vi "Motor Waveforms.vi"(10 "Log Data in":cluster{refnum<class "RDS State.lvclass">[]}[](array[cluster]), 11 "Log Header In":T1) -> (2 "Log Data out":cluster{refnum<class "RDS State.lvclass">[]}[](array[cluster]), 3 "Log Header Out":T1, 5 "STBD Motor WFs":waveform(dbl)[](array[waveform]), 7 "Port Motor WFs":waveform(dbl)[](array[waveform]))   [LabVIEW 2015, in "Log Waveform Processors.lvlib"]
uses:
  Log Waveform Processors.lvlib
  RDS State Tracker/RDS State/RDS State.lvclass
  Actors/RDS Logger Actor/RDS Logger Actor/RDS Logger Actor/Logger Header.ctl
  RDS State Tracker/RDS State/RDS State.lvclass/RDS State.ctl
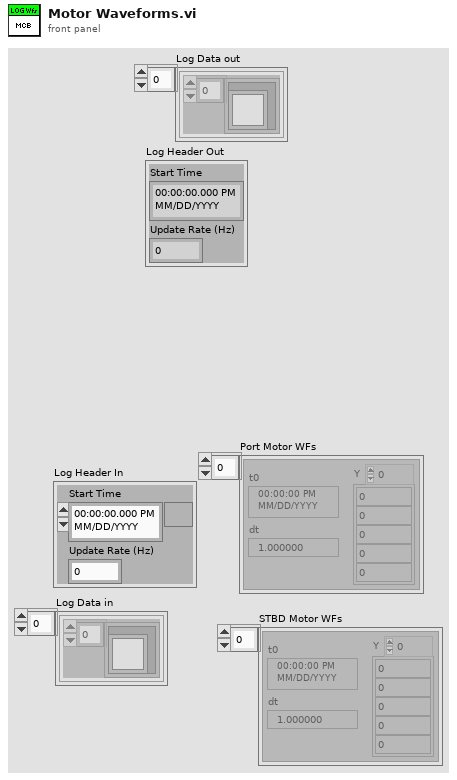
[diagram p1: front panel]
types:
  T1 = typedef "Log Waveform Processors.lvlib/Logger Header.ctl" = cluster{"Start Time":timestamp, "Update Rate (Hz)":dbl}
  T2 = typedef "RDS Child Messages.lvlib/MCB Motor Status.ctl" = cluster{"Motor Power":i16, "Motor Command":i16, "Battery Volts":sgl, "Battery Amps":sgl, "Motor Amps":sgl, "MCU Temp":i16, "Heatsink Temp":i16, "Fault Flags":u16, "StatusFlags":u16}
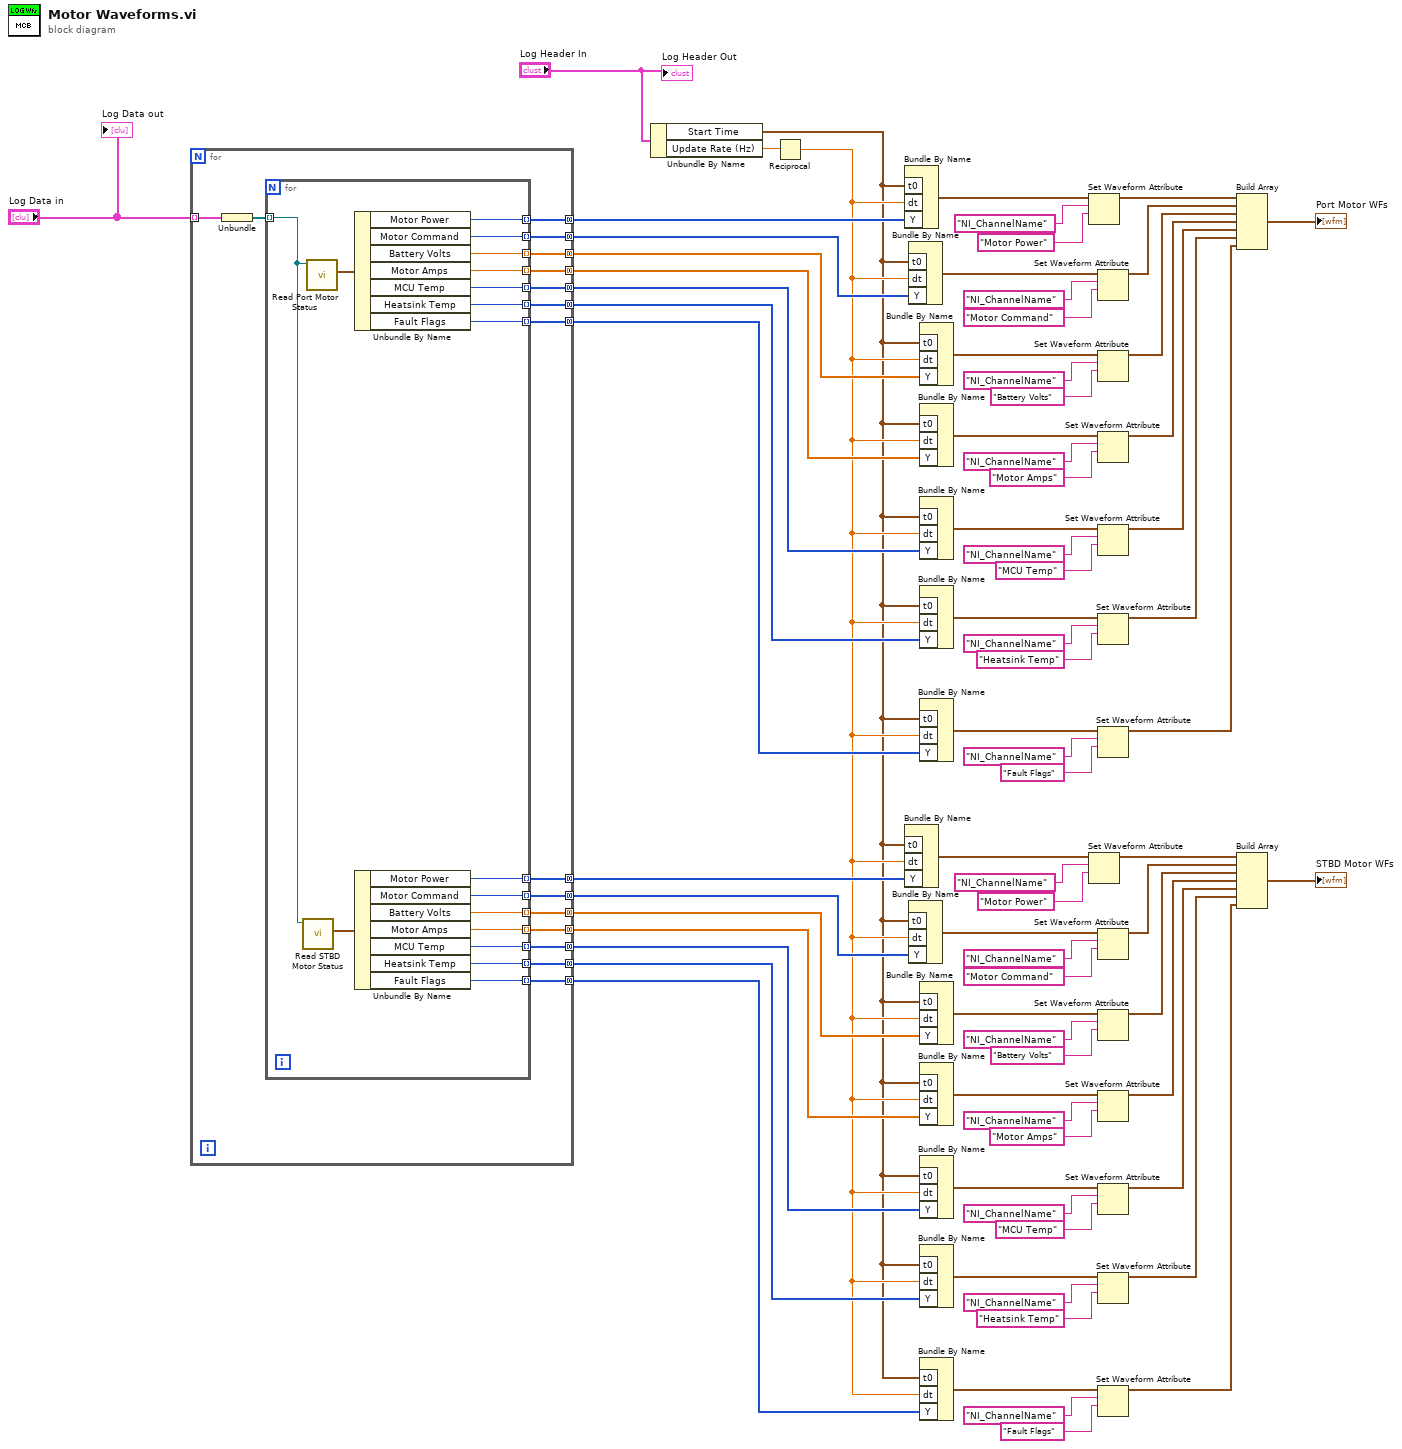
[diagram p0: block diagram]
diagram:
  n1 = for {
    tunnel: "Log Data in" -> [w93] mode=indexing
    tunnel: [w91] -> w47 mode=concatenating
    tunnel: [w90] -> w52 mode=concatenating
    tunnel: [w89] -> w53 mode=concatenating
    tunnel: [w88] -> w69 mode=concatenating
    tunnel: [w87] -> w70 mode=concatenating
    tunnel: [w86] -> w74 mode=concatenating
    tunnel: [w85] -> w40 mode=concatenating
    tunnel: [w78] -> w33 mode=concatenating
    tunnel: [w79] -> w28 mode=concatenating
    tunnel: [w80] -> w27 mode=concatenating
    tunnel: [w81] -> w11 mode=concatenating
    tunnel: [w82] -> w10 mode=concatenating
    tunnel: [w83] -> w6 mode=concatenating
    tunnel: [w84] -> w37 mode=concatenating
    n2 = Unbundle(w93) -> (w92:refnum<class "RDS State.lvclass">[])
    n3 = for {
      tunnel: w92 -> [w110] mode=indexing
      tunnel: [w108] -> w91 mode=indexing
      tunnel: [w107] -> w90 mode=indexing
      tunnel: [w106] -> w89 mode=indexing
      tunnel: [w105] -> w88 mode=indexing
      tunnel: [w104] -> w87 mode=indexing
      tunnel: [w103] -> w86 mode=indexing
      tunnel: [w102] -> w85 mode=indexing
      tunnel: [w95] -> w78 mode=indexing
      tunnel: [w96] -> w79 mode=indexing
      tunnel: [w97] -> w80 mode=indexing
      tunnel: [w98] -> w81 mode=indexing
      tunnel: [w99] -> w82 mode=indexing
      tunnel: [w100] -> w83 mode=indexing
      tunnel: [w101] -> w84 mode=indexing
      n4 = call "Read STBD Motor Status.vi"("RDS State in"=w110) -> ("STBD Motor"=w94:T2)  [unwired: 8 in, 2 out]
      n5 = call "Read Port Motor Status.vi"("RDS State in"=w110) -> ("Port Motor Data"=w109:T2)  [unwired: 8 in, 2 out]
      n6 = Unbundle By Name(w109) -> ("Motor Power"=w108:i16, "Motor Command"=w107:i16, "Battery Volts"=w106:sgl, "Motor Amps"=w105:sgl, "MCU Temp"=w104:i16, "Heatsink Temp"=w103:i16, "Fault Flags"=w102:u16)
      n7 = Unbundle By Name(w94) -> ("Motor Power"=w95:i16, "Motor Command"=w96:i16, "Battery Volts"=w97:sgl, "Motor Amps"=w98:sgl, "MCU Temp"=w99:i16, "Heatsink Temp"=w100:i16, "Fault Flags"=w101:u16)
    }
  }
  n8 = Unbundle By Name("Log Header In") -> ("Start Time"=w1:timestamp, "Update Rate (Hz)"=w44:dbl)
  n9 = Reciprocal(x=w44) -> (1/x=w2:dbl)
  n10 = Bundle By Name("t0"=w1, "dt"=w2, "Y"=w47) -> (w48:waveform(i16))  [unwired: 1 in]
  n11 = Bundle By Name("t0"=w1, "dt"=w2, "Y"=w33) -> (w32:waveform(i16))  [unwired: 1 in]
  n12 = Bundle By Name("t0"=w1, "dt"=w2, "Y"=w52) -> (w50:waveform(i16))  [unwired: 1 in]
  n13 = Bundle By Name("t0"=w1, "dt"=w2, "Y"=w28) -> (w30:waveform(i16))  [unwired: 1 in]
  n14 = Bundle By Name("t0"=w1, "dt"=w2, "Y"=w53) -> (w51:waveform(sgl))  [unwired: 1 in]
  n15 = Bundle By Name("t0"=w1, "dt"=w2, "Y"=w69) -> (w65:waveform(sgl))  [unwired: 1 in]
  n16 = Bundle By Name("t0"=w1, "dt"=w2, "Y"=w70) -> (w66:waveform(i16))  [unwired: 1 in]
  n17 = Bundle By Name("t0"=w1, "dt"=w2, "Y"=w74) -> (w73:waveform(i16))  [unwired: 1 in]
  n18 = Bundle By Name("t0"=w1, "dt"=w2, "Y"=w40) -> (w41:waveform(u16))  [unwired: 1 in]
  n19 = Bundle By Name("t0"=w1, "dt"=w2, "Y"=w27) -> (w29:waveform(sgl))  [unwired: 1 in]
  n20 = Bundle By Name("t0"=w1, "dt"=w2, "Y"=w11) -> (w15:waveform(sgl))  [unwired: 1 in]
  n21 = Bundle By Name("t0"=w1, "dt"=w2, "Y"=w10) -> (w14:waveform(i16))  [unwired: 1 in]
  n22 = Bundle By Name("t0"=w1, "dt"=w2, "Y"=w6) -> (w7:waveform(i16))  [unwired: 1 in]
  n23 = Bundle By Name("t0"=w1, "dt"=w2, "Y"=w37) -> (w36:waveform(u16))  [unwired: 1 in]
  n24 = Set Waveform Attribute(5:"Motor Power" ("name"), 6:"NI_ChannelName" ("name"), 7:w48) -> (3:w54:waveform(i16))  [unwired: 1 in, 2 out]
  n25 = Set Waveform Attribute(5:"Motor Power" ("name"), 6:"NI_ChannelName" ("name"), 7:w32) -> (3:w26:waveform(i16))  [unwired: 1 in, 2 out]
  n26 = Set Waveform Attribute(5:"Motor Command" ("name"), 6:"NI_ChannelName" ("name"), 7:w50) -> (3:w55:waveform(i16))  [unwired: 1 in, 2 out]
  n27 = Set Waveform Attribute(5:"Battery Volts" ("name"), 6:"NI_ChannelName" ("name"), 7:w51) -> (3:w56:waveform(sgl))  [unwired: 1 in, 2 out]
  n28 = Set Waveform Attribute(5:"Motor Amps" ("name"), 6:"NI_ChannelName" ("name"), 7:w65) -> (3:w75:waveform(sgl))  [unwired: 1 in, 2 out]
  n29 = Set Waveform Attribute(5:"MCU Temp" ("name"), 6:"NI_ChannelName" ("name"), 7:w66) -> (3:w76:waveform(i16))  [unwired: 1 in, 2 out]
  n30 = Set Waveform Attribute(5:"Heatsink Temp" ("name"), 6:"NI_ChannelName" ("name"), 7:w73) -> (3:w77:waveform(i16))  [unwired: 1 in, 2 out]
  n31 = Set Waveform Attribute(5:"Fault Flags" ("name"), 6:"NI_ChannelName" ("name"), 7:w41) -> (3:w39:waveform(u16))  [unwired: 1 in, 2 out]
  n32 = Set Waveform Attribute(5:"Motor Command" ("name"), 6:"NI_ChannelName" ("name"), 7:w30) -> (3:w25:waveform(i16))  [unwired: 1 in, 2 out]
  n33 = Set Waveform Attribute(5:"Battery Volts" ("name"), 6:"NI_ChannelName" ("name"), 7:w29) -> (3:w24:waveform(sgl))  [unwired: 1 in, 2 out]
  n34 = Set Waveform Attribute(5:"Motor Amps" ("name"), 6:"NI_ChannelName" ("name"), 7:w15) -> (3:w5:waveform(sgl))  [unwired: 1 in, 2 out]
  n35 = Set Waveform Attribute(5:"MCU Temp" ("name"), 6:"NI_ChannelName" ("name"), 7:w14) -> (3:w4:waveform(i16))  [unwired: 1 in, 2 out]
  n36 = Set Waveform Attribute(5:"Heatsink Temp" ("name"), 6:"NI_ChannelName" ("name"), 7:w7) -> (3:w3:waveform(i16))  [unwired: 1 in, 2 out]
  n37 = Set Waveform Attribute(5:"Fault Flags" ("name"), 6:"NI_ChannelName" ("name"), 7:w36) -> (3:w38:waveform(u16))  [unwired: 1 in, 2 out]
  n38 = Build Array(w54, w55, w56, w75, w76, w77, w39) -> (→"Port Motor WFs":waveform(sgl)[])
  n39 = Build Array(w26, w25, w24, w5, w4, w3, w38) -> (→"STBD Motor WFs":waveform(sgl)[])
  "Log Data out" <- "Log Data in"
  "Log Header Out" <- "Log Header In"
